vi "PreRunCTRL.vi"(8 "error in (no error)":errorcluster) -> (0 "error out":errorcluster)   [LabVIEW 2017, in "programControl.lvlib"]
doc: "This VI obtains the queue reference and notifier for the program control module.\n\nQueue = messages from all modules to the Program\nControl Module\n\nUser Event is used to send the 'start' message to \nall other modules."
uses:
  programControl.lvlib
  Queue/TypeDefs/queueFGVState.ctl
  StartUEFGV/TypeDefs/UEFGVcontrol.ctl
  SubVIs/FGVs/TypeDefs/DataFGVControl.ctl
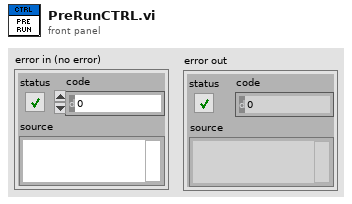
[diagram p1: front panel]
types:
  T1 = typedef "UEFGVcontrol.ctl" = enum16{"Create", "Get", "Destroy"}
  T2 = typedef "programControl.lvlib/queueFGVState.ctl" = enum16{"get", "set"}
  T3 = typedef "DataFGVControl.ctl" = enum16{"init", "Set DataOut", "Get DataOut", "Set DataIn", "Get DataIn"}
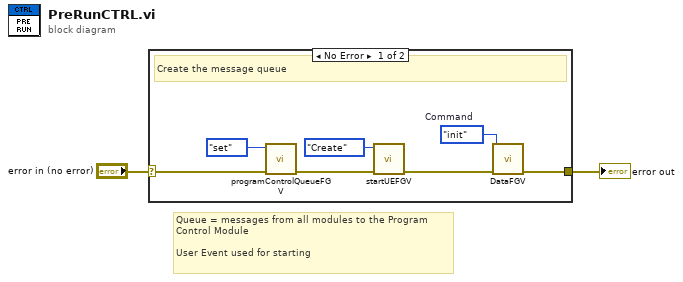
[diagram p0: block diagram]
diagram:
  # "Queue = messages from all modules to the Program\nControl Module\n\nUser Event used for starting"
  n1 = case shown="No Error" "error in (no error)" {
    selector: "error in (no error)" -> [w9 w10]
    tunnel: [w4 w10] -> w1
    frame No Error {
      w3 = DataFGVControl."init"  # Command
      # "Create the message queue"
      n2 = call "programControlQueueFGV.vi"("error in (no error)"=w9, 11:queueFGVState."set") -> ("error out"=w7:errorcluster)  [unwired: 8 in, 1 out]
      n3 = call "startUEFGV.vi"("error in (no error)"=w7, "Enum"=UEFGVcontrol."Create") -> ("error out"=w5:errorcluster)  [unwired: 8 in, 1 out]
      n4 = call "DataFGV.vi"("error in (no error)"=w5, "Command"=w3) -> ("error out"=w4:errorcluster)  [unwired: 7 in, 2 out]
    }
    frame Error {
    }
  }
  "error out" <- w1
